vi "Joint_Teleop.vi"(0 "Joystick_Out":T1, 1 "Visited_Disabled":bool) -> ()   [LabVIEW 2018]
uses:
  Utility_VIs/Joystick_Controls.ctl
  Subsytems/Intake_Joint/Intake_Joint_Notifier.ctl
  Subsytems/Intake_Joint/Intake_Joint_Control_Type.ctl
  Subsytems/Intake_Joint/Intake_Joint_Enum_States.ctl
  Global_Variables/LED_Globals.vi
  Global_Variables/Intake_Joint_Globals.vi
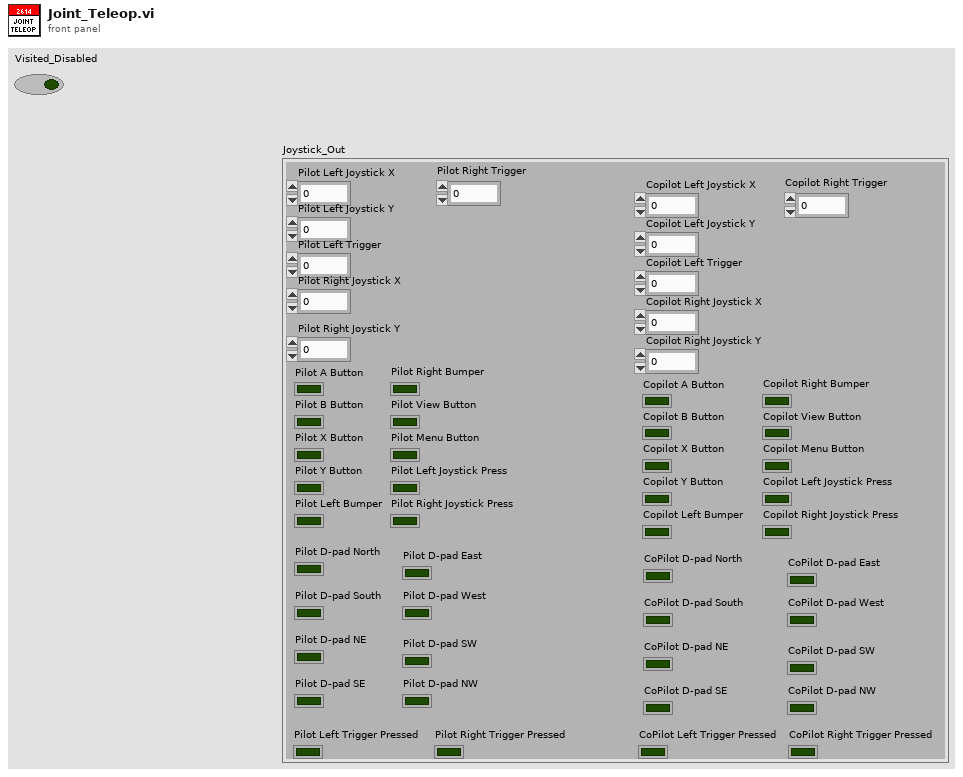
[diagram p1: front panel]
types:
  T1 = typedef "Joystick_Controls.ctl" = cluster{"Pilot Left Joystick X":dbl, "Pilot Left Joystick Y":dbl, "Pilot A Button":bool, "Pilot B Button":bool, "Pilot X Button":bool, "Pilot Y Button":bool, "Pilot Left Bumper":bool, "Pilot Right Bumper":bool, "Pilot View Button":bool, "Pilot Menu Button":bool, "Pilot Left Joystick Press":bool, "Pilot Right Joystick Press":bool, "Pilot Left Trigger":dbl, "Pilot Right Joystick X":dbl, "Pilot Right Joystick Y":dbl, "Pilot Right Trigger":dbl, "Copilot Left Joystick X":dbl, "Copilot Left Joystick Y":dbl, "Copilot A Button":bool, "Copilot B Button":bool, "Copilot X Button":bool, "Copilot Y Button":bool, "Copilot Left Bumper":bool, "Copilot Right Bumper":bool, "Copilot View Button":bool, "Copilot Menu Button":bool, "Copilot Left Joystick Press":bool, "Copilot Right Joystick Press":bool, "Copilot Left Trigger":dbl, "Copilot Right Joystick X":dbl, "Copilot Right Joystick Y":dbl, "Copilot Right Trigger":dbl, "Pilot D-pad North":bool, "Pilot D-pad South":bool, "Pilot D-pad East":bool, "Pilot D-pad West":bool, "Pilot D-pad NE ":bool, "Pilot D-pad SE":bool, "Pilot D-pad SW":bool, "Pilot D-pad NW":bool, "CoPilot D-pad North":bool, "CoPilot D-pad South":bool, "CoPilot D-pad East":bool, "CoPilot D-pad West":bool, "CoPilot D-pad NE":bool, "CoPilot D-pad SE":bool, "CoPilot D-pad SW":bool, "CoPilot D-pad NW":bool, "Pilot Left Trigger Pressed":bool, "Pilot Right Trigger Pressed":bool, "CoPilot Left Trigger Pressed":bool, "CoPilot Right Trigger Pressed":bool}
  T2 = typedef "Intake_Joint_Notifier.ctl" = cluster{"Intake_Joint_Control_Type":T3, "Manual_Joint_Up":bool, "Manual_Joint_Down":bool, "Low_Rocket":bool, "Mid_Rocket":bool, "High_Rocket":bool, "Cargo_Ship":bool, "Hatch_Floor":bool, "Cargo_Floor":bool, "HP_Hatch":bool, "HP_Cargo":bool, "Depot_Cargo":bool, "Stow":bool, "Intake_Mode":bool, "Set Position":T4}
  T3 = typedef "Intake_Joint_Control_Type.ctl" = enum16{"No_Op", "Manual_Joint_Up", "Manual_Joint_Down", "Manual_Position_Control", "Position_Control"}
  T4 = typedef "Intake_Joint_Enum_States.ctl" = enum16{"Current_Position", "High_Rocket_Hatch_Panel", "Mid_Rocket_Hatch_Panel", "Low_Rocket_Hatch_Panel", "Cargo_Ship_Hatch_Panel", "Loading_Station_Hatch_Panel", "Ground_Pickup_Hatch_Panel", "High_Rocket_Cargo", "Mid_Rocket_Cargo", "Low_Rocket_Cargo", "Cargo_Ship_Cargo", "Loading_Station_Cargo", "Ground_Pickup_Cargo", "Depot_Pickup_Cargo", "Stow_Cargo"}
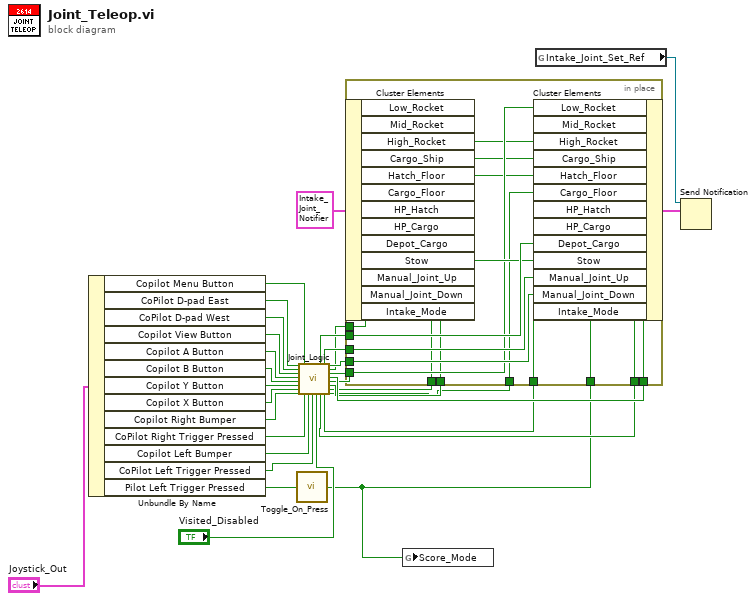
[diagram p0: block diagram]
diagram:
  n1 = Unbundle By Name("Joystick_Out") -> ("Copilot Menu Button"=w26:bool, "CoPilot D-pad East"=w25:bool, "CoPilot D-pad West"=w24:bool, "Copilot View Button"=w23:bool, "Copilot A Button"=w22:bool, "Copilot B Button"=w21:bool, "Copilot Y Button"=w20:bool, "Copilot X Button"=w19:bool, "Copilot Right Bumper"=w18:bool, "CoPilot Right Trigger Pressed"=w17:bool, "Copilot Left Bumper"=w16:bool, "CoPilot Left Trigger Pressed"=w15:bool, "Pilot Left Trigger Pressed"=w28:bool)
  n2 = call "Toggle_On_Press.vi"("Boolean"=w28) -> ("Boolean Out"=w1:bool)
  n3 = call "Joint_Logic.vi"("Manual_Up"=w25, "Manual_Down"=w24, "Stow"=w23, "Low_Rocket"=w22, "Mid_Rocket"=w21, "High_Rocket"=w20, "Cargo_Ship"=w19, "Hatch_Floor"=w18, "Depot_Cargo"=w26, "Cargo_Floor"=w17, "HP_Hatch"=w16, "HP_Cargo"=w15, "Visited_Disabled"="Visited_Disabled") -> ("Depot_Cargo_Out"=w13:bool, "HP_Cargo_Out"=w2:bool, "Manual_Up_Out"=w12:bool, "HP_Hatch_Out"=w3:bool, "Manual_Down_Out"=w11:bool, "Stow_Out"=w10:bool, "Low_Rocket_Out"=w9:bool, "Mid_Rocket_Out"=w8:bool, "High_Rocket_Out"=w7:bool, "Cargo_Ship_Out"=w6:bool, "Hatch_Floor_Out"=w5:bool, "Cargo_Floor_Out"=w4:bool)  [unwired: 3 in]
  n4 = in-place {
    in-place-border: w13 -> [w44]
    in-place-border: w12 -> [w43]
    in-place-border: w11 -> [w42]
    in-place-border: w10 -> [w41]
    in-place-border: w1 -> [w40]
    in-place-border: w9 -> [w39]
    in-place-border: w8 -> [w38]
    in-place-border: w7 -> [w37]
    in-place-border: w6 -> [w36]
    in-place-border: w5 -> [w35]
    in-place-border: w4 -> [w34]
    in-place-border: w3 -> [w33]
    in-place-border: w2 -> [w32]
    n5 = in-place-cluster #1(T2 {"Intake_Joint_Control_Type"=enum."No_Op", "Manual_Joint_Up"=FALSE, "Manual_Joint_Down"=FALSE, "Low_Rocket"=FALSE, "Mid_Rocket"=FALSE, "High_Rocket"=FALSE, "Cargo_Ship"=FALSE, "Hatch_Floor"=FALSE, "Cargo_Floor"=FALSE, "HP_Hatch"=FALSE, "HP_Cargo"=FALSE, "Depot_Cargo"=FALSE, "Stow"=FALSE, "Intake_Mode"=FALSE, "Set Position"=enum."High_Rocket_Hatch_Panel"} ("Intake_Joint_Notifier")) -> ()  [unwired: 13 out]
    n6 = in-place-cluster #1("Low_Rocket"=w39, "Mid_Rocket"=w38, "High_Rocket"=w37, "Cargo_Ship"=w36, "Hatch_Floor"=w35, "Cargo_Floor"=w34, "HP_Hatch"=w33, "HP_Cargo"=w32, "Depot_Cargo"=w44, "Stow"=w41, "Manual_Joint_Up"=w43, "Manual_Joint_Down"=w42, "Intake_Mode"=w40) -> (w31:T2)
  }
  n7 = global write "LED_Globals.vi" "Score_Mode"(w1) -> ()
  n8 = global read "Intake_Joint_Globals.vi" "Intake_Joint_Set_Ref"() -> (w29:refnum<notifier>)
  n9 = Send Notification(notification=w31, notifier=w29) -> ()  [unwired: 1 in, 2 out]
